vi "InitDaqList.vi"(8 "error in (no error)":errorcluster, 11 "DAQList in":refnum<class "DAQList.lvclass">) -> (0 "error out":errorcluster, 3 "DAQList out":refnum<class "DAQList.lvclass">)   [LabVIEW 2019, in "XCP_DaqDtoId.lvlib" / "DAQList.lvclass"]
uses:
  DAQList.lvclass
  DAQList.lvclass/DAQList.ctl
  DatabaseGeneration/SubVI_FilterDaqProcessorInfo.vi
  DatabaseGeneration/SubVI_FilterDaqResolutionInfo.vi
  XnetRead/InitMeaSplitInfo2.vi
  DatabaseGeneration/SubVI_ProcessMaxOdtEntrySize.vi
  DatabaseGeneration/SubVI_SetMeasProp.vi
  <vilib>/xnet/xnet.llb/XNET Create Session.vi
  <vilib>/xnet/xnet.llb/XNET Create Session (Frame Input Stream).vi
  <vilib>/xnet/xnet.llb/XNET Start.vi
  <vilib>/ECUMC/ECUMC.llb/MC DAQ List Initialize.vi
  <vilib>/ECUMC/ECUMC.llb/MC ECU Connect.vi
  <vilib>/ECUMC/ECUMC.llb/MC DAQ Start Stop.vi
  <vilib>/xnet/xnet.llb/XNET Read.vi
  <vilib>/xnet/xnet.llb/XNET Read (Frame CAN).vi
  <vilib>/xnet/xnet.llb/XNET Clear.vi
  <vilib>/ECUMC/ECUMC.llb/MC Get Property.vi
  <vilib>/ECUMC/ECUMC.llb/MC Get Prop XCP CRO Id.vi
  <vilib>/ECUMC/ECUMC.llb/MC Get Prop XCP DTO Id.vi
  <vilib>/ECUMC/ECUMC.llb/MC Get Prop XCP CAN IO Mode.vi
  <vilib>/ECUMC/ECUMC.llb/MC Get Prop XCP Baud Rate 64.vi
  <vilib>/ECUMC/ECUMC.llb/MC Get Prop XCP FD Baud Rate 64.vi
  <vilib>/xnet/xnet.llb/XNET Database Create Object.vi
  <vilib>/xnet/xnet.llb/XNET Database Create (Cluster).vi
  <vilib>/Utility/error.llb/Error Cluster From Error Code.vi
  <vilib>/xnet/xnet.llb/XNET Database Create (Frame).vi
  <vilib>/Utility/file.llb/Application Directory.vi
  <vilib>/xnet/xnet.llb/XNET Database Save.vi
  <vilib>/ECUMC/ECUMC.llb/MC Get Prop Meas Address.vi
  <vilib>/xnet/xnet.llb/XNET Database Create (Signal).vi
  <vilib>/xnet/xnet.llb/XNET Database Create (Subframe).vi
  <vilib>/ECUMC/ECUMC.llb/MC Get Prop Meas Data Type.vi
  <vilib>/xnet/xnet.llb/XNET Database Create (Dynamic Signal).vi
  <vilib>/ECUMC/ECUMC.llb/MC Get Prop Meas Comment.vi
  <vilib>/ECUMC/ECUMC.llb/MC Get Prop Meas Scaling Offset.vi
  <vilib>/ECUMC/ECUMC.llb/MC Get Prop Meas Scaling Factor.vi
  <vilib>/ECUMC/ECUMC.llb/MC Get Prop Meas Minimum.vi
  <vilib>/ECUMC/ECUMC.llb/MC Get Prop Meas Maximum.vi
  <vilib>/ECUMC/ECUMC.llb/MC Get Prop Meas Byte Order.vi
  <vilib>/ECUMC/ECUMC.llb/MC Get Prop Meas Unit.vi
  <vilib>/xnet/xnet.llb/XNET Create Session (Signal Input Waveform).vi
  TypeDef/Global.vi
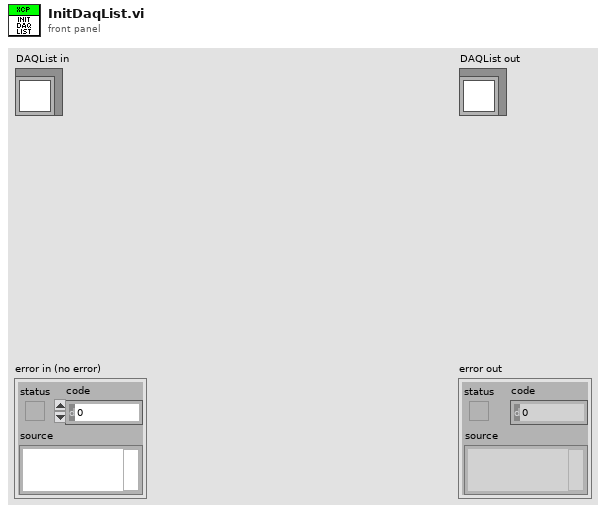
[diagram p1: front panel]
types:
  T1 = typedef "XNET Frame CAN.ctl" = cluster{"timestamp":timestamp, "payload":u8[], "identifier":u32, "type":T2, "extended?":bool, "echo?":bool}
  T2 = typedef "XNET Frame Type CAN.ctl" = u8
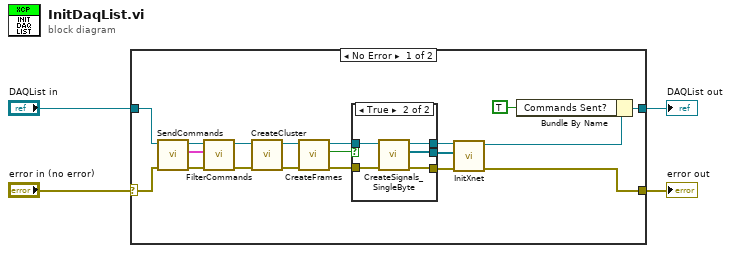
[diagram p0: block diagram]
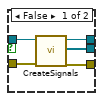
[diagram p2: hidden frame]
diagram:
  n1 = case shown="No Error" "error in (no error)" {
    selector: "error in (no error)" -> [w9 w35]
    tunnel: [w8 w35] -> w3
    tunnel: [w6 w34] -> w1
    tunnel: "DAQList in" -> [w10 w34]
    frame No Error {
      n2 = call "SendCommands.vi"("error in (no error)"=w9, "DAQList in"=w10) -> ("error out"=w23:errorcluster, "CAN Frames"=w21:T1[], "DAQList out"=w22:refnum<class "DAQList.lvclass">)  [unwired: 7 in]
      n3 = call "FilterCommands.vi"("error in (no error)"=w23, "CAN Frames"=w21, "DAQList in"=w22) -> ("error out"=w19:errorcluster, "DAQList out"=w20:refnum<class "DAQList.lvclass">)  [unwired: 7 in]
      n4 = call "CreateCluster.vi"("error in (no error)"=w19, "DAQList in"=w20) -> ("error out"=w17:errorcluster, "DAQList out"=w18:refnum<class "DAQList.lvclass">)  [unwired: 8 in]
      n5 = call "CreateFrames.vi"("error in (no error)"=w17, "DAQList in"=w18) -> ("error out"=w15:errorcluster, "DaqList_SingleByte"=w11:bool, "DAQList out"=w16:refnum<class "DAQList.lvclass">)  [unwired: 7 in]
      n6 = case shown="True" w11 {
        tunnel: w16 -> [w28 w33]
        tunnel: w15 -> [w27 w32]
        tunnel: [w26 w30] -> w14
        tunnel: [w25 w31] -> w13
        tunnel: [w24 w29] -> w12
        frame False {
          n7 = call "CreateSignals.vi"("error in (no error)"=w27, "DAQList in"=w28) -> ("error out"=w24:errorcluster, "Measurement Signals"=w25:refnum<k21>[], "DAQList out"=w26:refnum<class "DAQList.lvclass">)  [unwired: 7 in]
        }
        frame True {
          n8 = call "CreateSignals_SingleByte.vi"("error in (no error)"=w32, "DAQList in"=w33) -> ("error out"=w29:errorcluster, "Measurement Signals"=w31:refnum<k21>[], "DAQList out"=w30:refnum<class "DAQList.lvclass">)  [unwired: 7 in]
        }
      }
      n9 = call "InitXnet.vi"("error in (no error)"=w12, "Measurement Signals"=w13, "DAQList in"=w14) -> ("error out"=w8:errorcluster, "DAQList out"=w7:refnum<class "DAQList.lvclass">)  [unwired: 7 in]
      n10 = Bundle By Name(cluster=w7, "Commands Sent?"=TRUE) -> (w6:refnum<class "DAQList.lvclass">)
    }
    frame Error {
    }
  }
  "error out" <- w3
  "DAQList out" <- w1
